vi "NI9205_driver_OLD.vi"(6 "Method NI9205":T1, 8 "error in (no error)":errorcluster, 9 "Number of Samples":i32=100, 10 "Sample Rate":dbl=1000.0, 11 "Channels NI9205":tag="cDAQ1Mod3/ai0,cDAQ1Mod3/ai2") -> (0 "error out":errorcluster, 3 "Waveform Graph":waveform(dbl)[](graph))   [LabVIEW 2020]
uses:
  TYPEDEF/NI9205_TD_Method.ctl
  <vilib>/DAQmx/read.llb/DAQmx Read (Analog 1D Wfm NChan NSamp).vi
  <vilib>/DAQmx/miscellaneous.llb/DAQmx Fill In Error Info.vi
  <vilib>/Waveform/WDTOps.llb/WDT Get Waveform Time Array DBL.vi
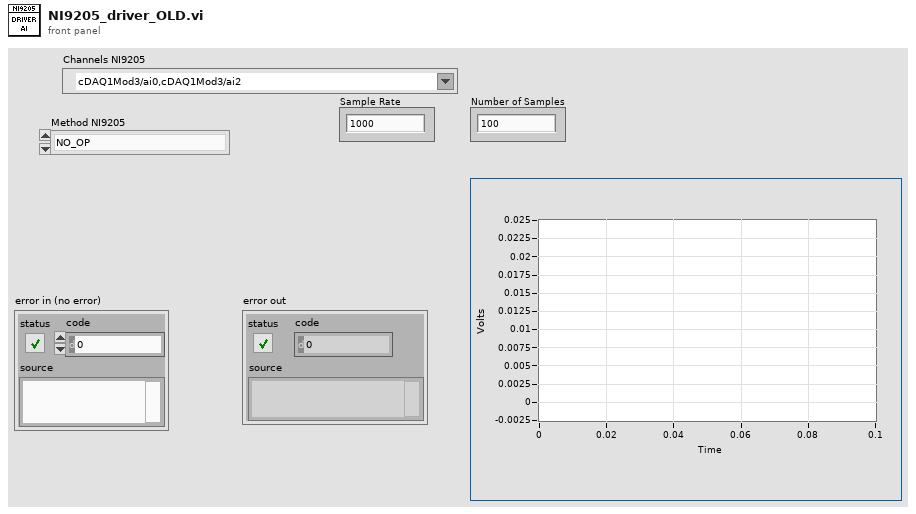
[diagram p1: front panel]
types:
  T1 = typedef "NI9205_TD_Method.ctl" = enum16{"NO_OP", "INIT", "SET", "GET", "CLOSE"}
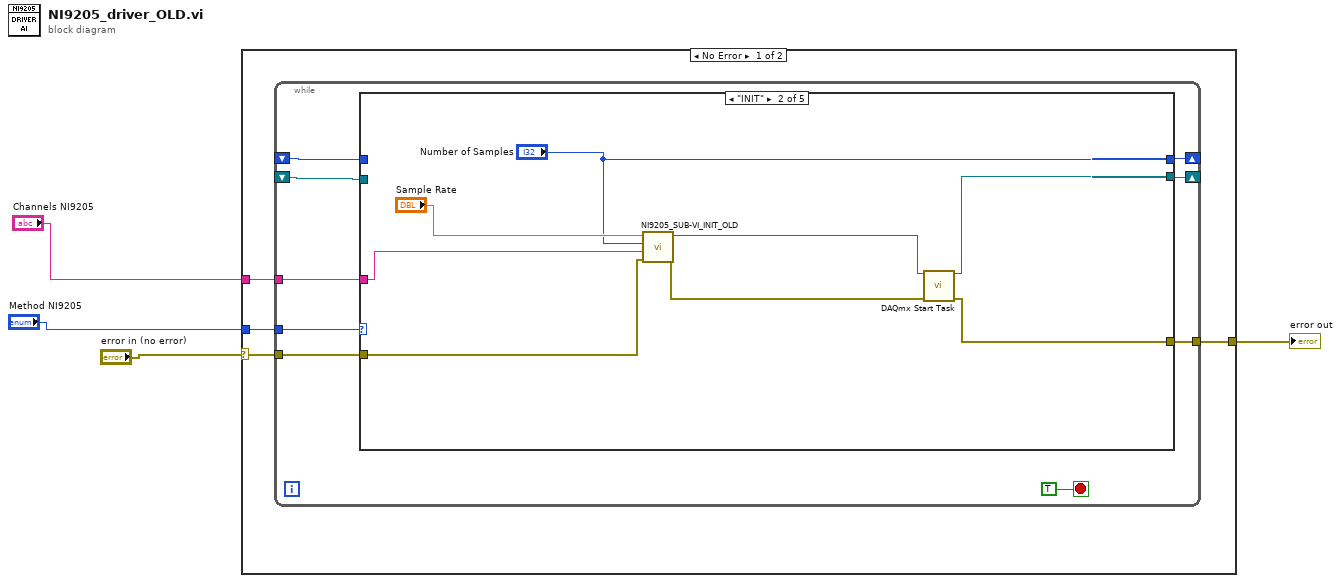
[diagram p0: block diagram]
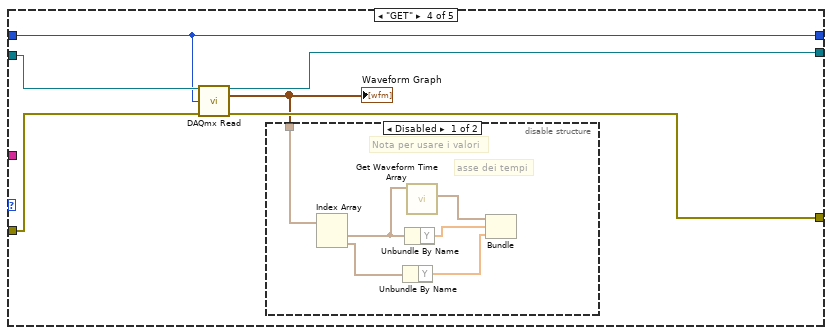
[diagram p4: hidden frame]
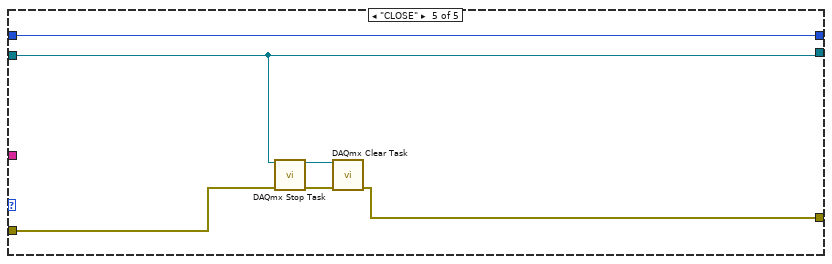
[diagram p6: hidden frame]
diagram:
  n1 = case shown="No Error" "error in (no error)" {
    selector: "error in (no error)" -> [w7 w50]
    tunnel: [w6 w50] -> w3
    tunnel: "Method NI9205" -> [w8 _]
    tunnel: "Channels NI9205" -> [w5 _]
    frame No Error {
      n2 = while {
        tunnel: w8 -> [w16]
        shift-right: [w15] -> _
        shift-left: _ -> [w11]
        shift-right: [w14] -> _
        shift-left: _ -> [w13]
        tunnel: w5 -> [w9]
        tunnel: w7 -> [w12]
        tunnel: [w10] -> w6
        stop <- TRUE stop-if-true
        n3 = case shown="\"INIT\"" w16 {
          tunnel: [w19 w25 w31 w34 w44] -> w15
          tunnel: [w20 "Number of Samples" w30 w36 w49] -> w14
          tunnel: w13 -> [w20 _ w30 w36 w49]
          tunnel: w12 -> [w18 w23 w29 w35 w46]
          tunnel: w11 -> [w19 _ w31 w37 w44]
          tunnel: [w18 w21 w29 w33 w45] -> w10
          tunnel: w9 -> [_ w22 _ _ _]
          frame "NO_OP", Default {
          }
          frame "INIT" {
            n4 = call "NI9205_SUB-VI_INIT_OLD.vi"("error in (no error)"=w23, "Channels NI9205"=w22, "Number of Samples"="Number of Samples", "Sample Rate"="Sample Rate") -> ("error out"=w27:errorcluster, "Refnum out"=w26:refnum<k21>)  [unwired: 6 in]
            n5 = call <vilib>:"DAQmx Start Task.vi"("task/channels in"=w26, "error in"=w27) -> ("task out"=w25:refnum<k21>, "error out"=w21:errorcluster)  [unwired: 12 in]
          }
          frame "SET" {
          }
          frame "GET" {
            n6 = call-poly <vilib>:"DAQmx Read.vi"("task/channels in"=w37, "number of samples per channel"=w36, "error in"=w35) -> ("task out"=w34:refnum<k21>, "data"=w32:waveform(dbl)[], "error out"=w33:errorcluster)  [unwired: 10 in]
            "Waveform Graph" <- w32
            n7 = disable-structure shown="Disabled" {
              disable-tunnel: w32 -> [w39 _]
              frame Disabled {
                # "asse dei tempi"
                # "Nota per usare i valori"
                n8 = Index Array(array=w39) -> (element #1=w38:waveform(dbl), element #2=w41:waveform(dbl))  [unwired: 2 in]
                n9 = Unbundle By Name(w41) -> ("Y"=w40:dbl[])
                n10 = Unbundle By Name(w38) -> ("Y"=w42:dbl[])
                n11 = call-poly <vilib>:"Get Waveform Time Array.vi"("waveform in"=w38) -> ("X array"=w43:timestamp[])  [unwired: 9 in, 1 out]
                n12 = Bundle("X array"=w43, "Y"=w42, "Y"=w40) -> ()  [unwired: 1 in, 1 out]
              }
              frame Enabled {
              }
            }
          }
          frame "CLOSE" {
            n13 = call <vilib>:"DAQmx Stop Task.vi"("task/channels in"=w44, "error in"=w46) -> ("task out"=w47:refnum<k21>, "error out"=w48:errorcluster)  [unwired: 12 in]
            n14 = call <vilib>:"DAQmx Clear Task.vi"("task in"=w47, "error in"=w48) -> ("error out"=w45:errorcluster)  [unwired: 13 in]
          }
        }
      }
    }
    frame Error {
    }
  }
  "error out" <- w3
